vi "adjust depth.vi"(6 "Current Depth":sgl, 7 "Read String Pot":bool, 9 "Depth Cluster":T1, 10 "Depth to \nbe Used \n(Feet)":sgl, 11 "Cluster in":refnum<vi>) -> (3 "Cluster out":T1)   [LabVIEW 2016]
uses:
  controls/Kpro hydraulic measurement cluster.ctl
  <vilib>/Analysis/baseanly.llb/Mean (DBL).vi
  <vilib>/Analysis/NI_AALBase.lvlib
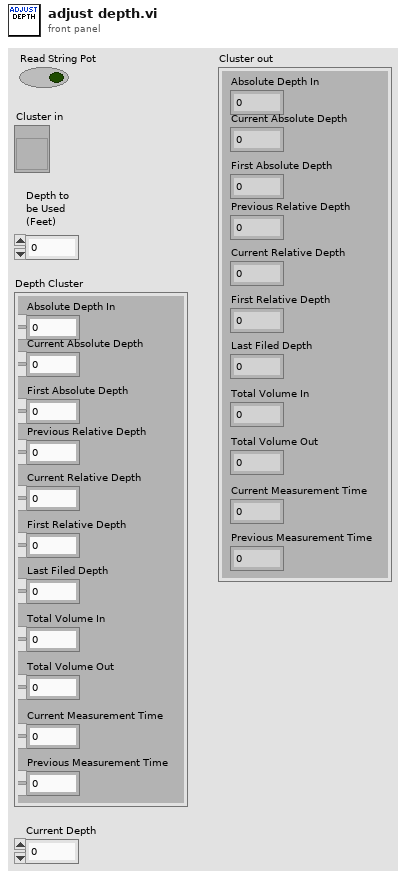
[diagram p1: front panel]
types:
  T1 = typedef "Kpro hydraulic measurement cluster.ctl" = cluster{"Absolute Depth In":dbl, "Current Absolute Depth":dbl, "First Absolute Depth":dbl, "Previous Relative Depth":dbl, "Current Relative Depth":dbl, "First Relative Depth":dbl, "Last Filed Depth":dbl, "Total Volume In":dbl, "Total Volume Out":dbl, "Current Measurement Time":dbl, "Previous Measurement Time":dbl}
  T2 = typedef "Sensor Physical Measurements.ctl" = cluster{"Uphole Pressure":dbl, "Flow":dbl, "Downhole Pressure":dbl, "Top String Pot":dbl, "String Pot":dbl, "Aux 1":dbl, "Aux 2":dbl, "Aux 3":dbl, "9V Monitor":dbl}
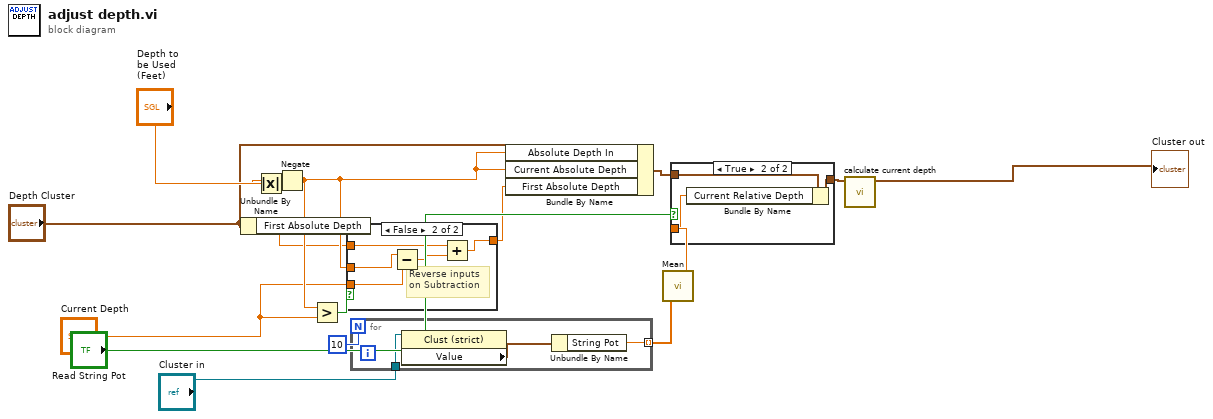
[diagram p0: block diagram]
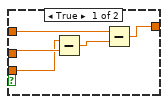
[diagram p3: hidden frame]
diagram:
  n1 = Unbundle By Name("Depth Cluster") -> ("First Absolute Depth"=w4:dbl)
  n2 = Absolute Value(x="Depth to \nbe Used \n(Feet)") -> (abs(x)=w12:sgl)
  n3 = Negate(x=w12) -> (-x=w13:sgl)
  n4 = Greater?(x=w13, y="Current Depth") -> (0:w7:bool)
  n5 = case shown="False" w7 {
    tunnel: [w21 w26] -> w3
    tunnel: w4 -> [w20 w25]
    tunnel: w13 -> [w18 w23]
    tunnel: "Current Depth" -> [w17 w22]
    frame True {
      n6 = Subtract(x=w17, y=w18) -> (x-y=w19:sgl)
      n7 = Subtract(x=w20, y=w19) -> (x-y=w21:dbl)
    }
    frame False {
      # "Reverse inputs \non Subtraction"
      n8 = Subtract(x=w23, y=w22) -> (x-y=w24:sgl)
      n9 = Add(x=w25, y=w24) -> (x+y=w26:dbl)
    }
  }
  n10 = for {
    N: 10 -> [_]
    tunnel: [w28] -> w10 mode=indexing
    tunnel: "Cluster in" -> [w27]
    n11 = property class="Clust (strict)"(reference=w27) -> ("Value"=w29:T2)  [unwired: 1 in, 2 out]
    n12 = Unbundle By Name(w29) -> ("String Pot"=w28:dbl)
  }
  n13 = Bundle By Name(cluster="Depth Cluster", "Absolute Depth In"=w13, "Current Absolute Depth"=w13, "First Absolute Depth"=w3) -> (w8:T1)
  n14 = call-poly <vilib>:"Mean.vi"("X"=w10) -> ("mean"=w16:dbl)  [unwired: 1 out]
  n15 = case shown="True" "Read String Pot" {
    tunnel: w8 -> [w30 w33]
    tunnel: [w30 w32] -> w9
    tunnel: w16 -> [_ w31]
    frame False {
    }
    frame True {
      n16 = Bundle By Name(cluster=w33, "Current Relative Depth"=w31) -> (w32:T1)
    }
  }
  n17 = call "calculate current depth.vi"("Cluster in"=w9) -> ("Cluster out"=→"Cluster out":T1)  [unwired: 10 in]
